vi "Terminate component.vi"(8 "error in (no error)":errorcluster, 10 "recipient":string, 11 "ServiceManager in":refnum<class "ServiceManager.lvclass">) -> (0 "error out":errorcluster, 3 "ServiceManager out":refnum<class "ServiceManager.lvclass">)   [LabVIEW 2012, in "ServiceManager.lvclass"]
uses:
  ServiceManager.lvclass
  <vilib>/Distrio/Murmex/TerminateMessage/TerminateMessage.lvclass
  ServiceManager.lvclass/ServiceManager.ctl
  <vilib>/Distrio/Murmex/Murmex/status_enum.ctl
  <vilib>/Distrio/Murmex/Murmex/Murmex.lvclass
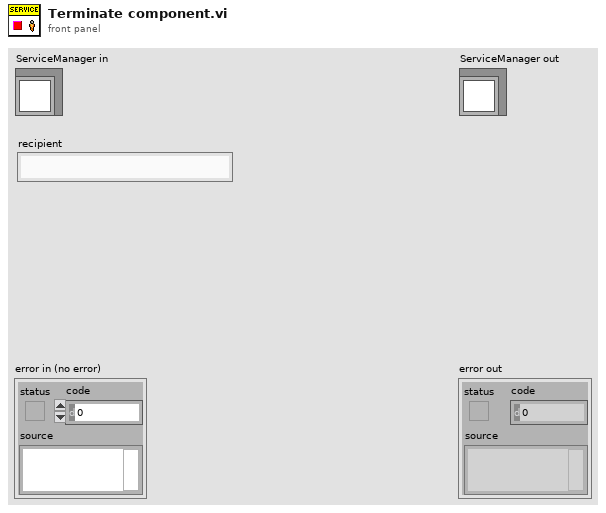
[diagram p1: front panel]
types:
  T1 = typedef "Murmex.lvlib/Murmex.lvclass/status_enum.ctl" = enum16{"ready", "warning", "error", "shutting down", "initialising"}
  T2 = typedef "ServiceManager.lvclass/loaded_components_cluster.ctl" = cluster{"component specification":T3, "booted?":bool, "status":T1, "last seen?":timestamp}
  T3 = typedef "Murmex.lvlib/Murmex.lvclass/component_specification_cluster.ctl" = cluster{"name":string, "language":string, "host name":string, "id":string}
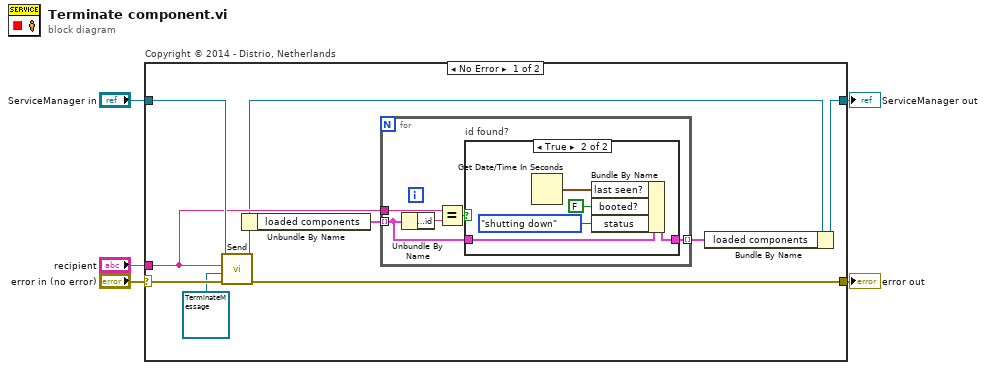
[diagram p0: block diagram]
diagram:
  n1 = case "Copyright © 2014 - Distrio, Netherlands" shown="No Error" "error in (no error)" {
    selector: "error in (no error)" -> [w7 w27]
    tunnel: [w14 w27] -> w4
    tunnel: [w8 w26] -> w2
    tunnel: "ServiceManager in" -> [w13 w26]
    tunnel: "recipient" -> [w11 _]
    frame No Error {
      n2 = call <vilib>:"Send.vi"("error in (no error)"=w7, "Message"=refnum<class "TerminateMessage.lvclass"> refnum ("TerminateMessage.lvclass"), "recipient"=w11, "Murmex in"=w13) -> ("error out"=w14:errorcluster, "Murmex out"=w9:refnum<class "ServiceManager.lvclass">)  [unwired: 6 in]
      n3 = Unbundle By Name(w9) -> ("loaded components"=w12:T2[])
      n4 = for {
        tunnel: w12 -> [w16] mode=indexing
        tunnel: w11 -> [w18]
        tunnel: [w15] -> w10 mode=indexing
        n5 = Unbundle By Name(w16) -> ("component specification.id"=w19:string)
        n6 = Equal?(x=w18, y=w19) -> (x = y?=w17:bool)
        n7 = case "id found?" shown="True" w17 {
          tunnel: w16 -> [w20 w25]
          tunnel: [w20 w22] -> w15
          frame False {
          }
          frame True {
            n8 = Get Date/Time In Seconds() -> (seconds since 1Jan1904=w21:timestamp)
            n9 = Bundle By Name(cluster=w25, "last seen?"=w21, "booted?"=FALSE, "status"=status_enum."shutting down") -> (w22:T2)
          }
        }
      }
      n10 = Bundle By Name(cluster=w9, "loaded components"=w10) -> (w8:refnum<class "ServiceManager.lvclass">)
    }
    frame Error {
    }
  }
  "error out" <- w4
  "ServiceManager out" <- w2
